vi "lorentzian from circle corners V5.vi"(7 "update z(inf)":enum16{"update z(inf)", "do not update z(inf)"}(ring)=enum."do not update z(inf)", 8 "omega map rameters in":T5={"frequency map method"=enum."less trivial", "2:window factor"=1, "left"=3.0, "right"=3.0, "omega"=3.0, "gamma"=3.0, "phi0"=3.0, "use points"=enum."decimated"}, 9 "circle corners in":T3={"z (-pi/2)"=-1.0311345636926572+0.5736824521422934i, "z(inf)"=-0.5200164984937075+1.0975277942502903i, "z (pi/2)"=-1.0311345636926572+0.5736824521422934i, "z center"=-0.5136528600391839+0.580046090596817i, "z(0)"=-0.5200164984937075+1.0975277942502903i, "radius"=-1.0311345636926572}, 10 "single fit parameters":T4={"number of 2D grid points"=200, "points after decimate"=93, "points before decimate"=4107, "decimation threshold"=1, "normalization factor"=0.005102552585135461, "complex region scale factor "=3.0, "normalized z"=array[4107 elements], "decimated z"=[0.4086999416726234+0.27653084474993667i, 0.4043675507393041+0.27187411611263035i, 0.3992152446406012+0.2866690148407477i, 0.38987681782092737+0.2796656705890701i, 0.3885478852115913+0.2853795752756981i, 0.37424677933088596+0.2916882969614883i, 0.36630586164105544+0.3013059695755191i, 0.3572225626966358+0.30157620929133466i, 0.3591607134412589+0.29870858500022546i, 0.34526037877213844+0.31577462619112134i, 0.3445358699361499+0.31396964671575356i, 0.34153004285372884+0.3154426636204338i, 0.335540381789013+0.3324302726540888i, 0.3288084132766795+0.33071696133989303i, 0.31551809708239975+0.34888246168069326i, 0.31398233630231437+0.34672841403398275i, 0.3124324305476661+0.34491167614050133i, 0.30168334846436345+0.36141080840589246i, 0.29960036161555575+0.3644765501140444i, 0.2787745634489416+0.3734961799530281i, 0.28247402044526565+0.37556030547495095i, 0.2654426354393931+0.38646722616569107i, 0.26085737469193576+0.39138156461276274i, 0.25158048144751116+0.4029098233705838i, 0.2437503606544421+0.40592983109982583i, 0.23659257658410568+0.4136463545042213i, 0.2208696574903446+0.4218755314447385i, 0.2037668036192148+0.4366037031685101i, 0.19187442018415896+0.438624011369513i, 0.17720511497204394+0.4432070269259341i, 0.1662607775835308+0.45453571196556497i, 0.1493802753732626+0.4639049582412799i, 0.1254511476775962+0.46748653333915113i, 0.1033303949534509+0.47813813399968913i, 0.0760179586599686+0.49136482745797033i, 0.03938352213850839+0.49341366586536217i, -0.008082261483109483+0.4963810216710412i, -0.060527992100659955+0.4985012896125286i, -0.13210308037505086+0.48328769389477994i, -0.2164964209072893+0.4579329803588853i, -0.31155150322000724+0.3898071876364797i, -0.41080908136967736+0.2764696089956603i, -0.47571311945822425+0.07542461980130123i, -0.43238189747242073-0.1750684238452788i, -0.2500583167802815-0.4029543655469544i, -0.003067977826097106-0.5014987103874714i, 0.19664864922046021-0.46877458226049556i, 0.3264592182464339-0.3841076764481272i, 0.39139158572573973-0.3045223037293669i, 0.4298267647472987-0.23258711184176573i, 0.4548604103609155-0.16798872385217029i, 0.46806747869399146-0.11764777517569555i, 0.47115569073873115-0.07926649929358924i, 0.46837628871708364-0.03694571328228424i, 0.47270651062714336-0.003809525374196055i, 0.47273283266207666+0.022081820056540025i, 0.4667717445305655+0.04127384443801294i, 0.46226887863084654+0.06320802982448562i, 0.4583729632879457+0.0875130923779392i, 0.4520889996996694+0.10406128252952807i, 0.45832267413717875+0.11311681771625329i, 0.4516869799167576+0.12298372020551539i, 0.4446055090004313+0.13178584688391243i, 0.44366854423885344+0.14231364306558697i, 0.4363006495505189+0.15757450828036026i, 0.42643994503455573+0.16593716221082852i, 0.42351872677287233+0.18339449448440692i, 0.41720623232577153+0.1988615890082908i, 0.41113704427571934+0.2125100714557952i, 0.40332364427545486+0.21990096302627865i, 0.4049190262834987+0.2293473262438519i, 0.39563214482126824+0.2405824404108469i, 0.38970786326899837+0.23506354711018443i, 0.3899681508881921+0.24823254471928627i, 0.3859413642570831+0.2582459848210299i, 0.3749803175874859+0.26059699274280157i, 0.3738379694867003+0.2718717578317005i, 0.35827051260491116+0.278162192718538i, 0.34435024044548757+0.2904452656920766i, 0.3297983655271314+0.29946214288730544i, 0.3299532953040057+0.30170168613834203i, 0.3258372999664237+0.31568274442045086i, 0.314591109715885+0.31037433654935476i, 0.31309403813828984+0.31627103049926253i, 0.29999544340655704+0.32049208568773396i, 0.29938213309261735+0.3149537822739577i, 0.28417087915090317+0.32544691504728024i, 0.29058669132467924+0.33251923664556715i, 0.2826528975116781+0.33032835058892424i, 0.2688413815997774+0.32858284064475973i, 0.2698123346444453+0.33078816617434537i, 0.25412663124852986+0.33157104396518056i, 0.2536781441982096+0.32875576565267184i], "decimated omega"=[2044.092, 2044.152, 2049.044, 2049.226, 2050.635, 2055.528, 2059.695, 2061.97, 2062.494, 2065.051, 2065.594, 2065.634, 2066.48, 2066.641, 2067.003, 2067.024, 2067.044, 2067.225, 2067.245, 2067.386, 2067.406, 2067.467, 2067.527, 2067.567, 2067.587, 2067.607, 2067.648, 2067.688, 2067.708, 2067.728, 2067.748, 2067.769, 2067.789, 2067.809, 2067.829, 2067.849, 2067.869, 2067.889, 2067.909, 2067.93, 2067.95, 2067.97, 2067.99, 2068.01, 2068.03, 2068.05, 2068.071, 2068.091, 2068.111, 2068.131, 2068.151, 2068.171, 2068.191, 2068.211, 2068.232, 2068.252, 2068.272, 2068.292, 2068.332, 2068.352, 2068.373, 2068.393, 2068.413, 2068.433, 2068.473, 2068.513, 2068.594, 2068.675, 2068.755, 2068.876, 2068.896, 2069.097, 2069.138, 2069.319, 2069.5, 2070.003, 2070.305, 2072.097, 2076.99, 2083.956, 2084.298, 2088.204, 2092.07, 2093.237, 2099.136, 2101.653, 2106.988, 2108.257, 2109.545, 2114.699, 2115.505, 2119.934, 2121.464], "omega in window"=array[4107 elements], "z in window"=array[4107 elements], "data center"=-0.0014901433980738042-0.0014987103874714112i, "inverse"=[], "linear "=[], "omega around"=[], "whatever plot"=[]}, 11 "cursor window":T1={"left"=2378.60310421286, "right "=2421.6740576496672, "center"=2421.6740576496672, "window"=2421.6740576496672, "cursors"=[], "relative"=0, "absolute"=0, "plot ref"=refnum, "Cursor List"=[], "fixed vertical offset"=2421.6740576496672, "vertical offset"=2421.6740576496672, "horizontal offset"=2421.6740576496672, "default window frac"=2421.6740576496672}) -> (0 "omega map rameters  out":T5={"frequency map method"=enum."less trivial", "2:window factor"=1, "left"=3.0, "right"=3.0, "omega"=3.0, "gamma"=3.0, "phi0"=3.0, "use points"=enum."decimated"}, 1 "circle corners out":T3={"z (-pi/2)"=-1.0311345636926572+0.5736824521422934i, "z(inf)"=-0.5200164984937075+1.0975277942502903i, "z (pi/2)"=-1.0311345636926572+0.5736824521422934i, "z center"=-0.5136528600391839+0.580046090596817i, "z(0)"=-0.5200164984937075+1.0975277942502903i, "radius"=-1.0311345636926572}, 3 "lorentzian out":T6={"Amplitude"=-1.0311345636926572, "omega(0)"=-1.0311345636926572, "Gamma"=-1.0311345636926572, "phi"=-1.0311345636926572, "Q"=-1.0311345636926572, "Norm  Ampl"=-1.0311345636926572, "z (inf)"=-1.0311345636926572+0.0i})   [LabVIEW 2010]
uses:
  <vilib>/Analysis/NI_AALPro.lvlib
  <vilib>/gmath/NI_Gmath.lvlib
  <vilib>/gmath/NumericalOptimization/Nonlinear Curve Fit LM.vi
  <vilib>/gmath/NumericalOptimization/LM model function reference.ctl
  <vilib>/Analysis/6fits.llb/Curve Fitting Criteria.ctl
  <vilib>/gmath/NumericalOptimization/Nonlinear Curve Fit LM formula string.vi
  circle corners.ctl
  lorentzian.ctl
  omega map parameters.ctl
  single fit parameters.ctl
  cursor winow.ctl
  <vilib>/Utility/miscctls.llb/LVCursorListTypeDef.ctl
panel:
  in  "lorentzian dummy 3":T6={"Amplitude"=-1.0311345636926572, "omega(0)"=-1.0311345636926572, "Gamma"=-1.0311345636926572, "phi"=-1.0311345636926572, "Q"=-1.0311345636926572, "Norm  Ampl"=-1.0311345636926572, "z (inf)"=-1.0311345636926572+0.0i}
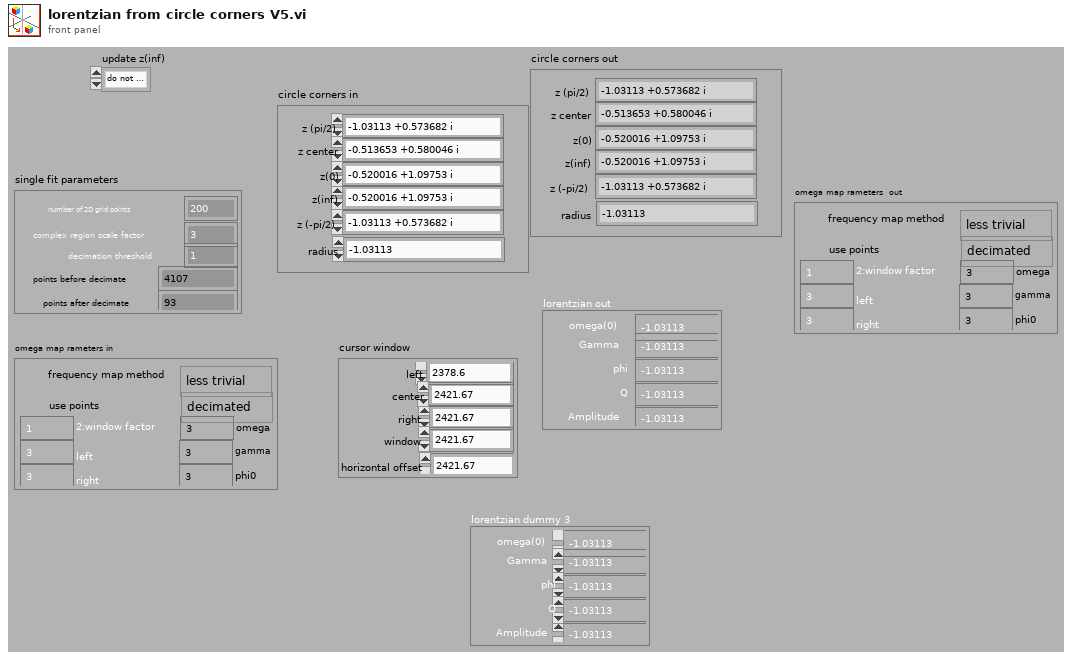
[diagram p1: front panel]
types:
  T1 = typedef "cursor winow.ctl" = cluster{"left":dbl, "right ":dbl, "center":dbl, "window":dbl, "cursors":i32[], "relative":i32, "absolute":i32, "plot ref":refnum<vi>, "Cursor List":T2, "fixed vertical offset":dbl, "vertical offset":dbl, "horizontal offset":dbl, "default window frac":dbl}
  T2 = typedef "LVCursorListTypeDef.ctl" = cluster{"Name":string, "Color":u32, "Style":u8, "Point Style":u8, "Name Visible":bool, "Allow Drag":bool, "Cursor Mode":u32, "Plot":i32, "Index":i32, "Position":cluster{"X":dbl, "Y":dbl}, "X Scale":u32, "Y Scale":u32, "Watch Plots":i32[], "Watch All Plots":bool, "Plot Area":i32, "Label Offset":cluster{"X":dbl, "Y":dbl}}[]
  T3 = typedef "circle corners.ctl" = cluster{"z (-pi/2)":cdb, "z(inf)":cdb, "z (pi/2)":cdb, "z center":cdb, "z(0)":cdb, "radius":dbl}
  T4 = typedef "single fit parameters.ctl" = cluster{"number of 2D grid points":i32, "points after decimate":i32, "points before decimate":i32, "decimation threshold":i32, "normalization factor":dbl, "complex region scale factor ":dbl, "normalized z":cdb[], "decimated z":cdb[], "decimated omega":dbl[], "omega in window":dbl[], "z in window":cdb[], "data center":cdb, "inverse":cdb[], "linear ":cdb[], "omega around":dbl[], "whatever plot":cluster{"omega":dbl[], dbl[]}[]}
  T5 = typedef "omega map parameters.ctl" = cluster{"frequency map method":enum16{"simple", "less trivial", "super fancy", "geometry"}, "2:window factor":i32, "left":dbl, "right":dbl, "omega":dbl, "gamma":dbl, "phi0":dbl, "use points":enum16{"all in window", "decimated"}}
  T6 = typedef "lorentzian.ctl" = cluster{"Amplitude":dbl, "omega(0)":dbl, "Gamma":dbl, "phi":dbl, "Q":dbl, "Norm  Ampl":dbl, "z (inf)":cdb}
  T7 = enum16{"simple method one", "not so simple method two", "super method three"}
  T8 = enum16{"simple", "less trivial", "super fancy", "geometry"}
  T9 = typedef "NI_Gmath.lvlib/LM model function reference.ctl" = refnum<vi>
  T10 = cluster{"model":string, "Parameters":string[], "x":string}
  T11 = cluster{"decimated omega":dbl[], "Unwrapped Phase":dbl[]}
  T12 = cluster{"decimated omega":dbl[], "best nonlinear fit":dbl[]}
  T13 = cluster{"decimated omega":dbl[], "best nonlinear fit":dbl[]}[]
  T14 = typedef "NI_AALPro.lvlib/Curve Fitting Criteria.ctl" = u16
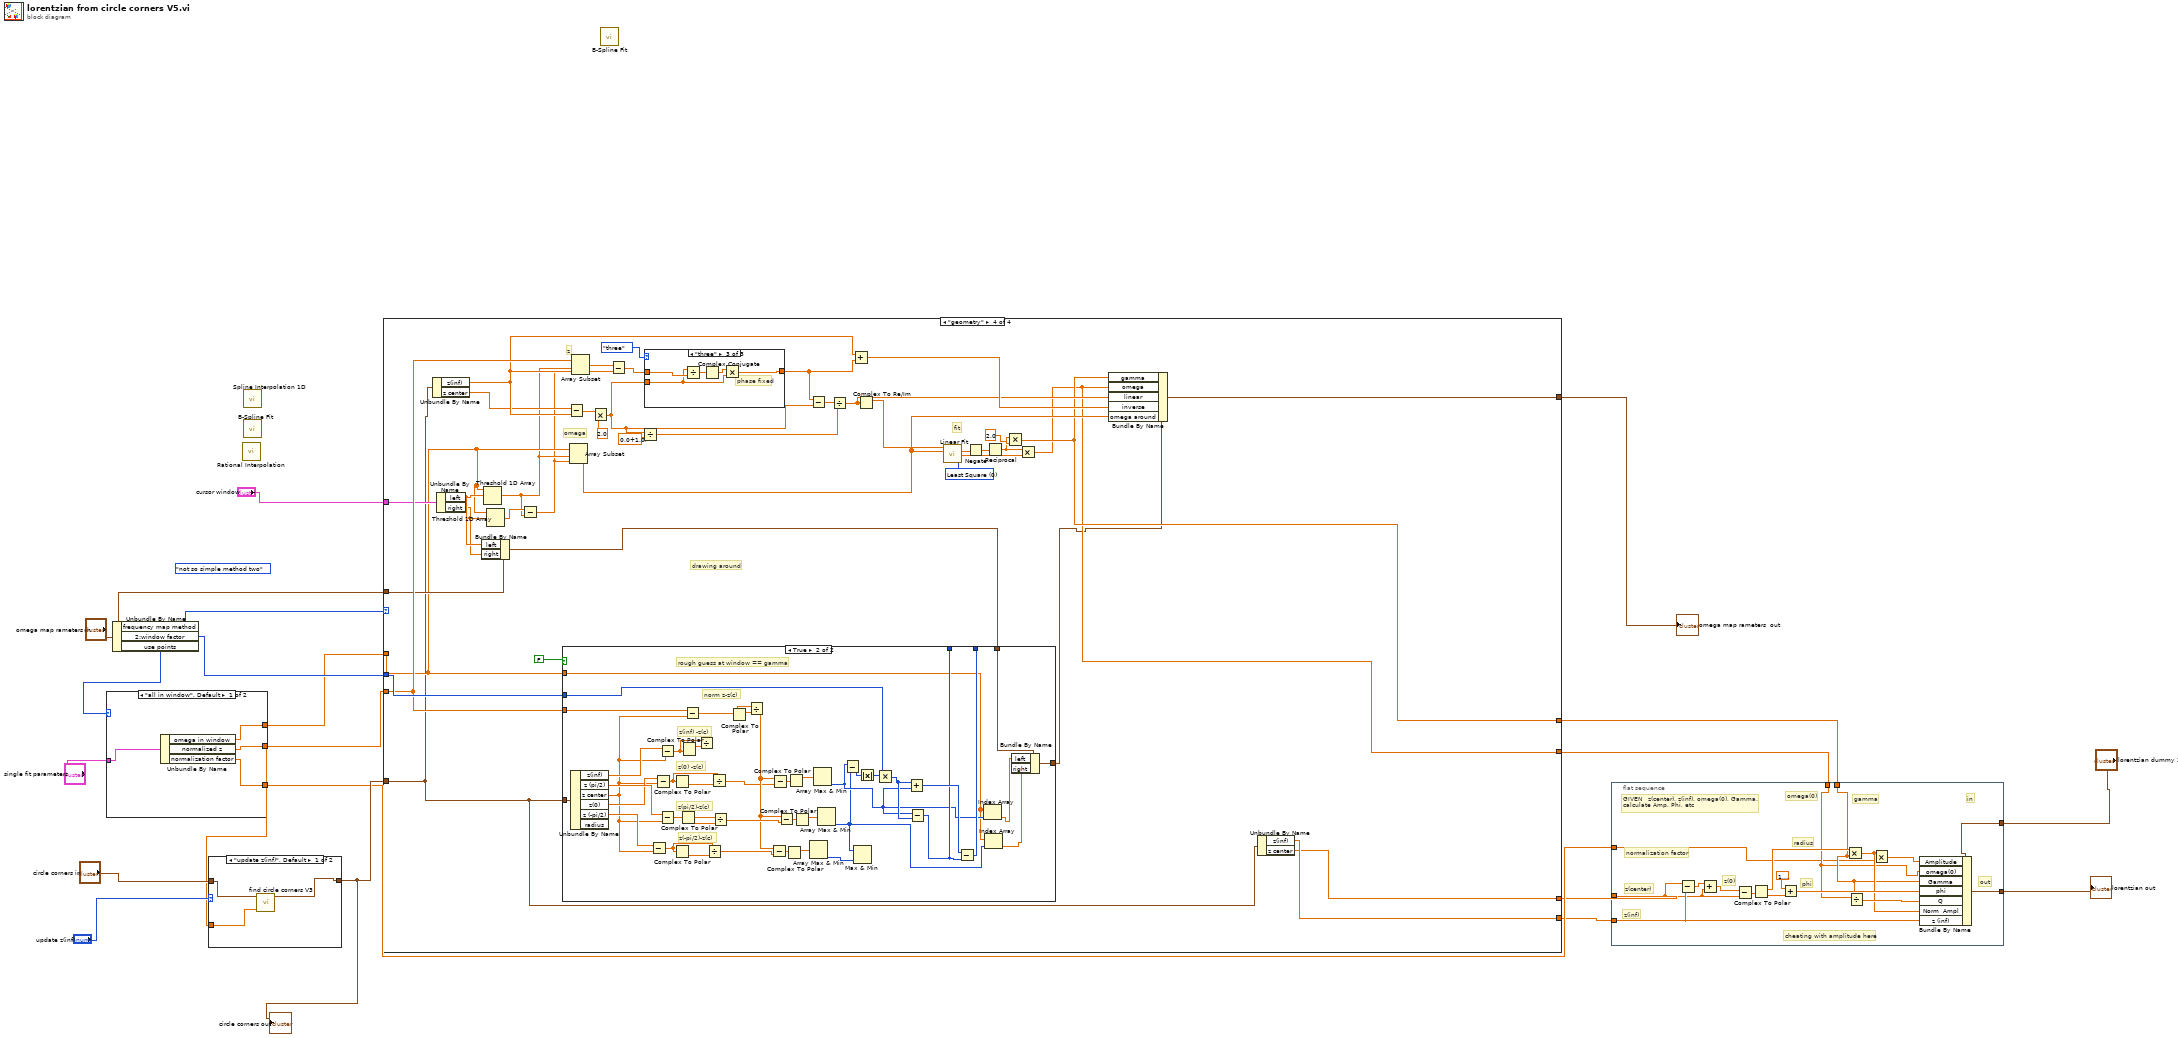
[diagram p0: block diagram]
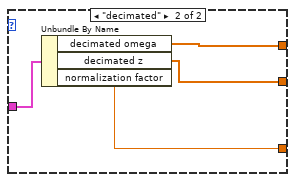
[diagram p3: hidden frame]
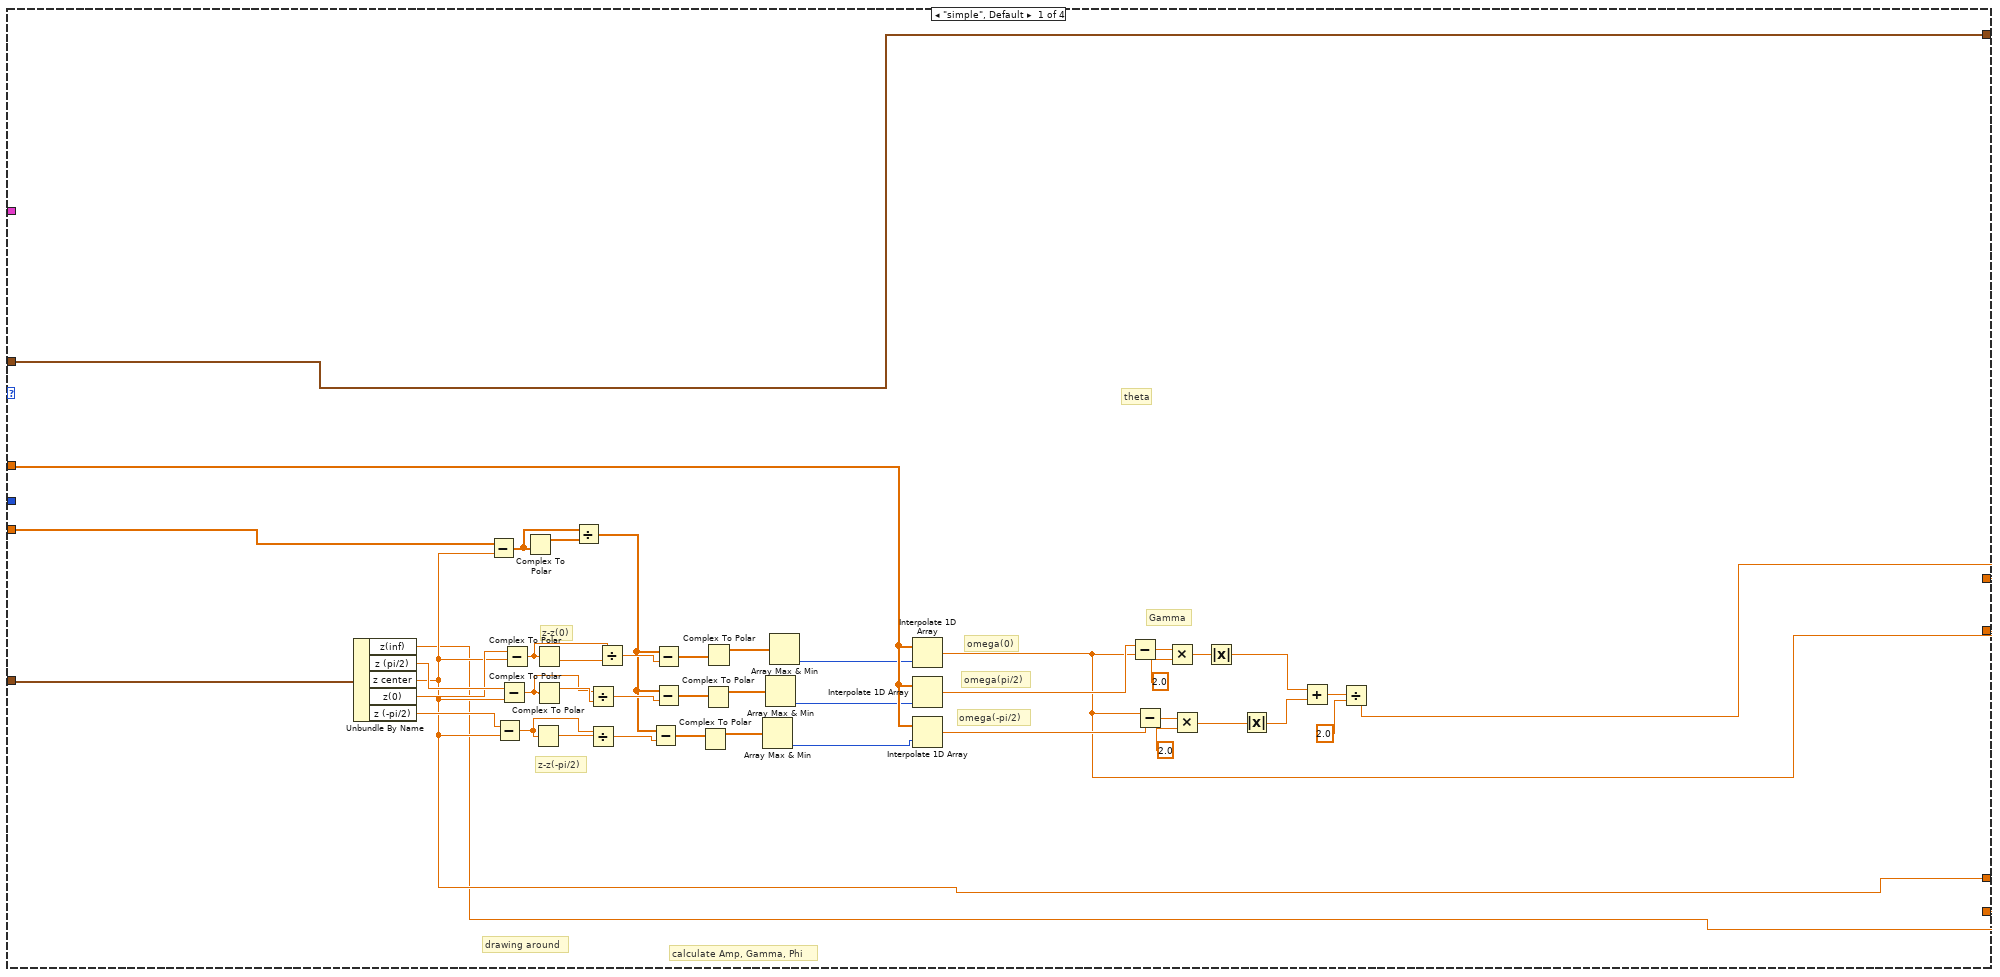
[diagram p4: hidden frame]
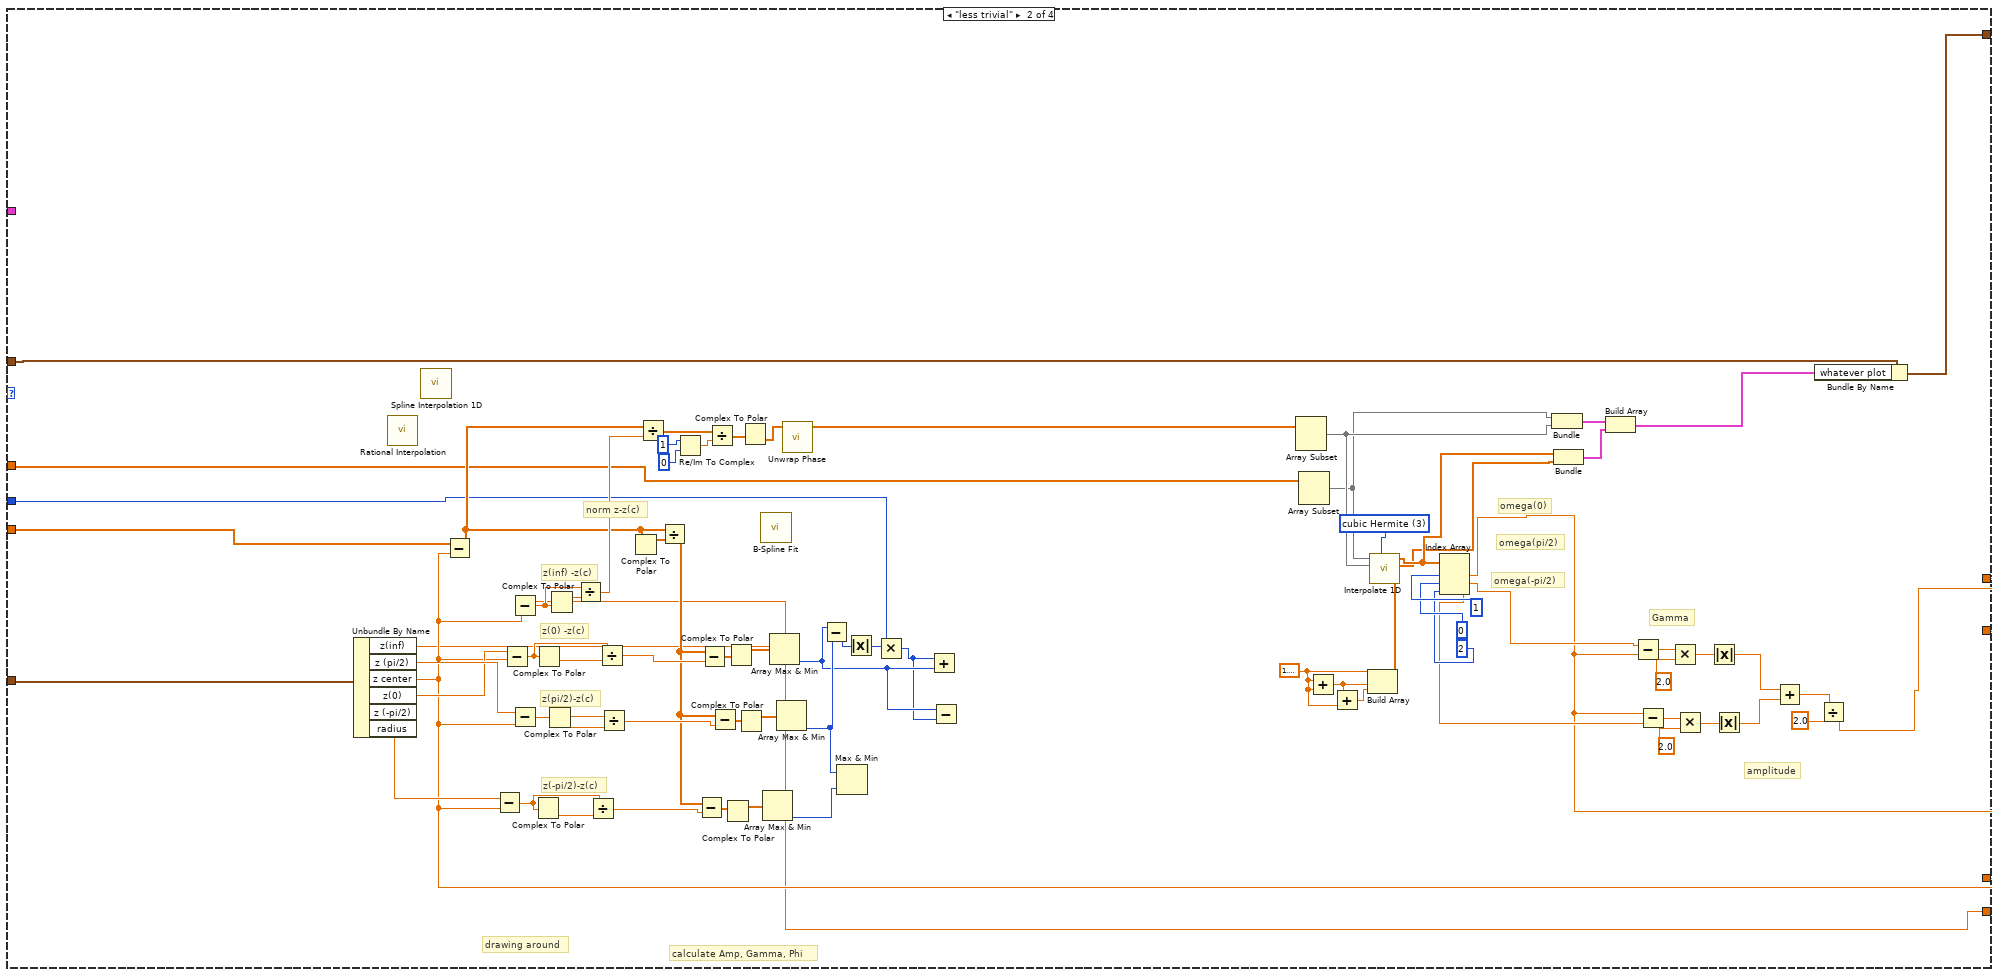
[diagram p5: hidden frame]
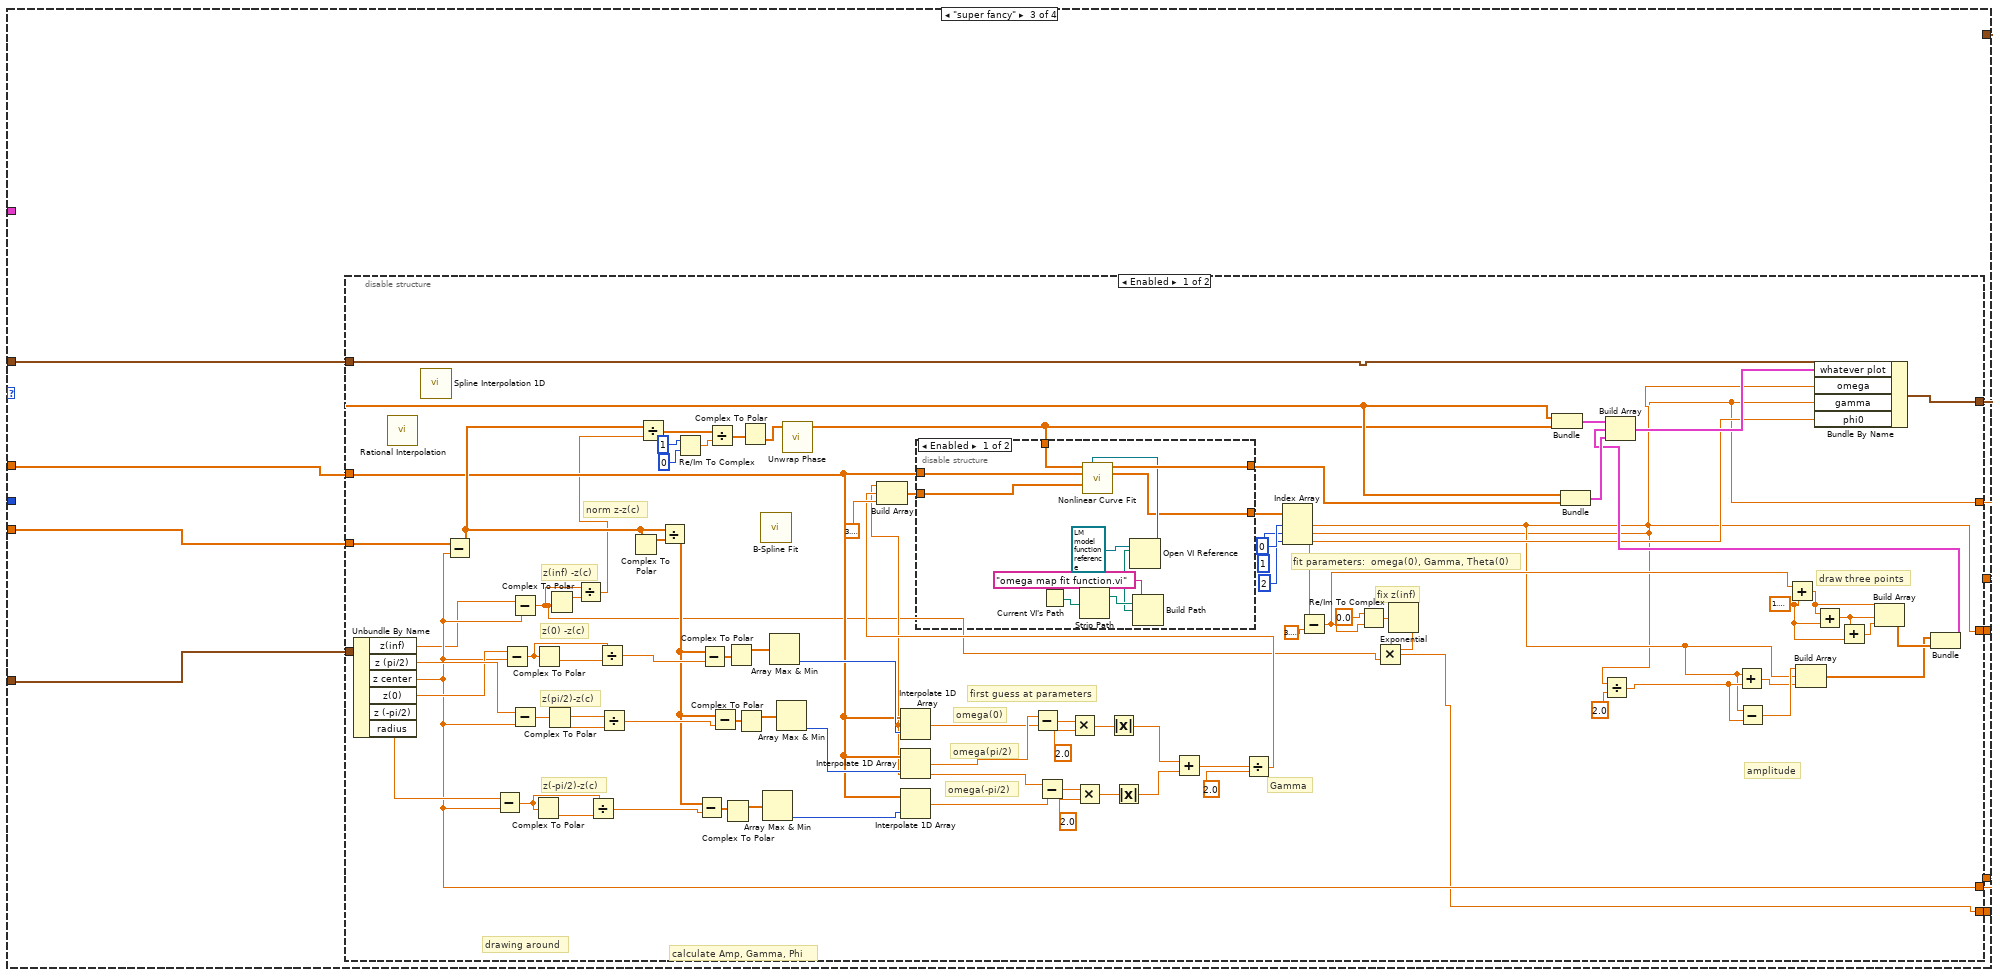
[diagram p6: hidden frame]
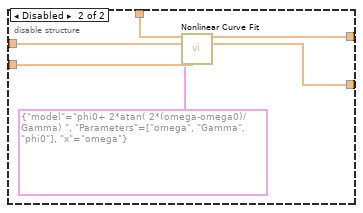
[diagram p7: hidden frame]
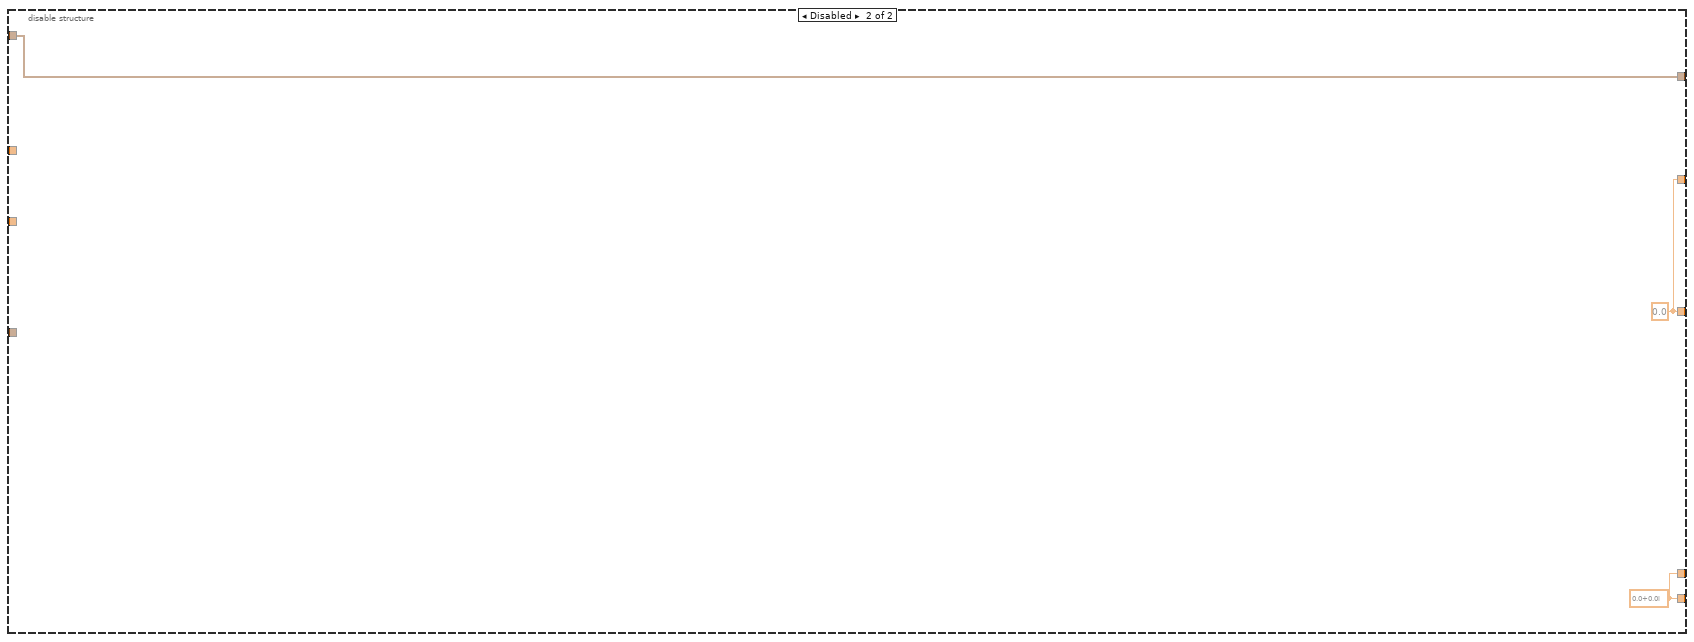
[diagram p8: hidden frame]
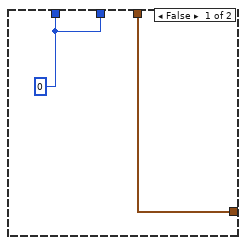
[diagram p9: hidden frame]
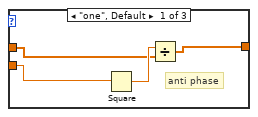
[diagram p10: hidden frame]
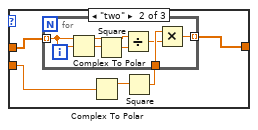
[diagram p11: hidden frame]
diagram:
  (unwired) T7."not so simple method two"
  n1 = Unbundle By Name("omega map rameters in") -> ("frequency map method"=w19:T8, "2:window factor"=w16:i32, "use points"=w13:enum16{"all in window", "decimated"})
  n2 = case shown="\"all in window\", Default" w13 {
    tunnel: "single fit parameters" -> [w23 w27]
    tunnel: [w22 w26] -> w14
    tunnel: [w21 w25] -> w10
    tunnel: [w20 w24] -> w4
    frame "all in window", Default {
      n3 = Unbundle By Name(w23) -> ("omega in window"=w22:dbl[], "normalized z"=w21:cdb[], "normalization factor"=w20:dbl)
    }
    frame "decimated" {
      n4 = Unbundle By Name(w27) -> ("decimated omega"=w26:dbl[], "decimated z"=w25:cdb[], "normalization factor"=w24:dbl)
    }
  }
  n5 = case shown="\"update z(inf)\", Default" "update z(inf)" {
    tunnel: [w29 w31] -> w9
    tunnel: "circle corners in" -> [w30 w31]
    tunnel: w10 -> [w28 _]
    frame "update z(inf)", Default {
      n6 = call "find circle corners V3.vi"("z"=w28, "circle corners in"=w30) -> ("circle corners out"=w29:T3)  [unwired: 9 in]
    }
    frame "do not update z(inf)" {
    }
  }
  "circle corners out" <- w9
  n7 = call <vilib>:"Rational Interpolation.vi"() -> ()  [unwired: 3 in, 3 out]
  n8 = call <vilib>:"Spline Interpolation 1D.vi"() -> ()  [unwired: 9 in, 3 out]
  n9 = call <vilib>:"B-Spline Fit.vi"() -> ()  [unwired: 12 in, 4 out]
  n10 = case shown="\"geometry\"" w19 {
    tunnel: w9 -> [w71 w146 w158 w264]
    tunnel: w10 -> [w70 w145 w157 w297]
    tunnel: w14 -> [w59 w105 w155 w270]
    tunnel: "omega map rameters in" -> [w36 w80 w154 w275]
    tunnel: [w36 w87 w156 w304] -> w17
    tunnel: w16 -> [_ w86 _ w303]
    tunnel: [w34 w78 w152 w281] -> w6
    tunnel: [w35 w79 w153 w280] -> w5
    tunnel: [w33 w77 w151 w265] -> w3
    tunnel: [w32 w76 w150 w266] -> w2
    tunnel: "cursor window" -> [_ _ _ w277]
    frame "simple", Default {
      # "z-z(-pi/2)"
      # "z-z(0)"
      # "omega(-pi/2)"
      # "omega(pi/2)"
      # "omega(0)"
      # "theta"
      # "Gamma"
      # "calculate Amp, Gamma, Phi"
      # "drawing around"
      n11 = Unbundle By Name(w71) -> ("z(inf)"=w32:cdb, "z (pi/2)"=w69:cdb, "z center"=w33:cdb, "z(0)"=w68:cdb, "z (-pi/2)"=w67:cdb)
      n12 = Subtract(x=w70, y=w33) -> (x-y=w51:cdb[])
      n13 = Subtract(x=w67, y=w33) -> (x-y=w54:cdb)
      n14 = Subtract(x=w69, y=w33) -> (x-y=w53:cdb)
      n15 = Subtract(x=w68, y=w33) -> (x-y=w58:cdb)
      n16 = Complex To Polar(r * e^(i*theta)=w51) -> (r=w52:dbl[])  [unwired: 1 out]
      n17 = Complex To Polar(r * e^(i*theta)=w54) -> (r=w56:dbl)  [unwired: 1 out]
      n18 = Complex To Polar(r * e^(i*theta)=w58) -> (r=w57:dbl)  [unwired: 1 out]
      n19 = Complex To Polar(r * e^(i*theta)=w53) -> (r=w55:dbl)  [unwired: 1 out]
      n20 = Divide(x=w51, y=w52) -> (x/y=w47:cdb[])
      n21 = Divide(x=w53, y=w55) -> (x/y=w49:cdb)
      n22 = Divide(x=w54, y=w56) -> (x/y=w48:cdb)
      n23 = Divide(x=w58, y=w57) -> (x/y=w50:cdb)
      n24 = Subtract(x=w47, y=w48) -> (x-y=w45:cdb[])
      n25 = Subtract(x=w47, y=w50) -> (x-y=w46:cdb[])
      n26 = Subtract(x=w47, y=w49) -> (x-y=w44:cdb[])
      n27 = Complex To Polar(r * e^(i*theta)=w45) -> (r=w41:dbl[])  [unwired: 1 out]
      n28 = Complex To Polar(r * e^(i*theta)=w44) -> (r=w42:dbl[])  [unwired: 1 out]
      n29 = Complex To Polar(r * e^(i*theta)=w46) -> (r=w43:dbl[])  [unwired: 1 out]
      n30 = Array Max & Min(array=w41) -> (min index (indices)=w40:i32)  [unwired: 3 out]
      n31 = Array Max & Min(array=w42) -> (min index (indices)=w39:i32)  [unwired: 3 out]
      n32 = Array Max & Min(array=w43) -> (min index (indices)=w38:i32)  [unwired: 3 out]
      n33 = Interpolate 1D Array(1:w38, 2:w59) -> (0:w35:dbl)
      n34 = Interpolate 1D Array(1:w39, 2:w59) -> (0:w72:dbl)
      n35 = Interpolate 1D Array(1:w40, 2:w59) -> (0:w60:dbl)
      n36 = Subtract(x=w72, y=w35) -> (x-y=w75:dbl)
      n37 = Subtract(x=w35, y=w60) -> (x-y=w66:dbl)
      n38 = Multiply(x=w75, y=2.0) -> (x*y=w73:dbl)
      n39 = Multiply(x=w66, y=2.0) -> (x*y=w64:dbl)
      n40 = Absolute Value(x=w73) -> (abs(x)=w63:dbl)
      n41 = Absolute Value(x=w64) -> (abs(x)=w37:dbl)
      n42 = Add(x=w63, y=w37) -> (x+y=w62:dbl)
      n43 = Divide(x=w62, y=2.0) -> (x/y=w34:dbl)
    }
    frame "less trivial" {
      w101 = 1.5707963267948966
      w103 = 3 items=["nearest", "linear", "spline", "cubic Hermite", "Lagrange"] ("method")
      # "z(pi/2)-z(c)"
      # "z(inf) -z(c)"
      # "norm z-z(c)"
      # "z(-pi/2)-z(c)"
      # "z(0) -z(c)"
      # "omega(-pi/2)"
      # "omega(pi/2)"
      # "omega(0)"
      # "amplitude"
      # "Gamma"
      # "calculate Amp, Gamma, Phi"
      # "drawing around"
      n44 = Unbundle By Name(w146) -> ("z(inf)"=w76:cdb, "z (pi/2)"=w144:cdb, "z center"=w77:cdb, "z(0)"=w143:cdb, "z (-pi/2)"=w142:cdb)  [unwired: 1 out]
      n45 = call <vilib>:"Rational Interpolation.vi"() -> ()  [unwired: 3 in, 3 out]
      n46 = call <vilib>:"Spline Interpolation 1D.vi"() -> ()  [unwired: 9 in, 3 out]
      n47 = Subtract(x=w145, y=w77) -> (x-y=w114:cdb[])
      n48 = Subtract(x=w142, y=w77) -> (x-y=w132:cdb)
      n49 = Subtract(x=w143, y=w77) -> (x-y=w135:cdb)
      n50 = Subtract(x=w76, y=w77) -> (x-y=w118:cdb)
      n51 = Subtract(x=w144, y=w77) -> (x-y=w131:cdb)
      n52 = Complex To Polar(r * e^(i*theta)=w132) -> (r=w133:dbl)  [unwired: 1 out]
      n53 = Complex To Polar(r * e^(i*theta)=w135) -> (r=w134:dbl)  [unwired: 1 out]
      n54 = Complex To Polar(r * e^(i*theta)=w131) -> (r=w107:dbl)  [unwired: 1 out]
      n55 = Complex To Polar(r * e^(i*theta)=w118) -> (r=w119:dbl)  [unwired: 1 out]
      n56 = Divide(x=w118, y=w119) -> (x/y=w117:cdb)
      n57 = Divide(x=w132, y=w133) -> (x/y=w127:cdb)
      n58 = Divide(x=w135, y=w134) -> (x/y=w129:cdb)
      n59 = Divide(x=w131, y=w107) -> (x/y=w128:cdb)
      n60 = Complex To Polar(r * e^(i*theta)=w114) -> (r=w130:dbl[])  [unwired: 1 out]
      n61 = Divide(x=w114, y=w117) -> (x/y=w110:cdb[])
      n62 = Divide(x=w114, y=w130) -> (x/y=w116:cdb[])
      n63 = Re/Im To Complex(1:0, 2:1) -> (0:w112:cdb)
      n64 = Subtract(x=w116, y=w127) -> (x-y=w125:cdb[])
      n65 = Subtract(x=w116, y=w129) -> (x-y=w126:cdb[])
      n66 = Divide(x=w110, y=w112) -> (x/y=w113:cdb[])
      n67 = Subtract(x=w116, y=w128) -> (x-y=w124:cdb[])
      n68 = Complex To Polar(r * e^(i*theta)=w125) -> (r=w121:dbl[])  [unwired: 1 out]
      n69 = Complex To Polar(r * e^(i*theta)=w126) -> (r=w123:dbl[])  [unwired: 1 out]
      n70 = Complex To Polar(r * e^(i*theta)=w124) -> (r=w122:dbl[])  [unwired: 1 out]
      n71 = Complex To Polar(r * e^(i*theta)=w113) -> (theta=w108:dbl[])  [unwired: 1 out]
      n72 = call <vilib>:"B-Spline Fit.vi"() -> ()  [unwired: 12 in, 4 out]
      n73 = Array Max & Min(array=w121) -> (min index (indices)=w106:i32)  [unwired: 3 out]
      n74 = Array Max & Min(array=w123) -> (min index (indices)=w90:i32)  [unwired: 3 out]
      n75 = Array Max & Min(array=w122) -> (min index (indices)=w93:i32)  [unwired: 3 out]
      n76 = call <vilib>:"Unwrap Phase.vi"("Phase"=w108) -> ("Unwrapped Phase"=w104:dbl[])  [unwired: 9 in, 1 out]
      n77 = Subtract(x=w90, y=w93) -> (x-y=w92:i32)
      n78 = Max & Min(x=w93, y=w106) -> ()  [unwired: 2 out]
      n79 = Absolute Value(x=w92) -> (abs(x)=w91:i32)
      n80 = Multiply(x=w91, y=w86) -> (x*y=w89:i32)
      n81 = Add(x=w89, y=w90) -> ()  [unwired: 1 out]
      n82 = Subtract(x=w90, y=w89) -> ()  [unwired: 1 out]
      n83 = Array Subset(array=w104) -> (w95:dbl[])  [unwired: 2 in]
      n84 = Array Subset(array=w105) -> (w94:dbl[])  [unwired: 2 in]
      n85 = Add(x=w101, y=w101) -> (x+y=w102:dbl)
      n86 = Add(x=w102, y=w101) -> (x+y=w100:dbl)
      n87 = Build Array(w101, w102, w100) -> (w99:dbl[])
      n88 = call <vilib>:"Interpolate 1D.vi"("method"=w103, "xi"=w99, "X"=w95, "Y"=w94) -> ("xi used"=w84:dbl[], "yi"=w85:dbl[])  [unwired: 5 in, 1 out]
      n89 = Index Array(array=w85, index #1=1, index #2=0, index #3=2) -> (element #1=w79:dbl, element #2=w82:dbl, element #3=w81:dbl)
      n90 = Bundle(w94, w95) -> (w115:cluster{dbl[], dbl[]})  [unwired: 1 in]
      n91 = Bundle("yi"=w85, "xi used"=w84) -> (w83:cluster{"yi":dbl[], "xi used":dbl[]})  [unwired: 1 in]
      n92 = Build Array(w115, w83) -> (w88:cluster{"yi":dbl[], "xi used":dbl[]}[])
      n93 = Subtract(x=w82, y=w79) -> (x-y=w149:dbl)
      n94 = Subtract(x=w79, y=w81) -> (x-y=w141:dbl)
      n95 = Multiply(x=w149, y=2.0) -> (x*y=w147:dbl)
      n96 = Multiply(x=w141, y=2.0) -> (x*y=w139:dbl)
      n97 = Absolute Value(x=w147) -> (abs(x)=w138:dbl)
      n98 = Absolute Value(x=w139) -> (abs(x)=w120:dbl)
      n99 = Add(x=w138, y=w120) -> (x+y=w137:dbl)
      n100 = Bundle By Name(cluster=w80, "whatever plot"=w88) -> (w87:T5)
      n101 = Divide(x=w137, y=2.0) -> (x/y=w78:dbl)
    }
    frame "super fancy" {
      n102 = disable-structure shown="Enabled" {
        disable-tunnel: w158 -> [w243 _]
        disable-tunnel: w157 -> [w242 _]
        disable-tunnel: [w211 w263] -> w156
        disable-tunnel: w155 -> [w193 _]
        disable-tunnel: w154 -> [w191 w263]
        disable-tunnel: [w163 w261] -> w153
        disable-tunnel: [w162 w261] -> w152
        disable-tunnel: [w161 w262] -> w151
        disable-tunnel: [w159 w262] -> w150
        frame Enabled {
          w167 = 1.5707963267948966
          # "fix z(inf)"
          # "fit parameters:  omega(0), Gamma, Theta(0)"
          # "draw three points"
          # "first guess at parameters"
          # "omega(-pi/2)"
          # "omega(pi/2)"
          # "omega(0)"
          # "Gamma"
          # "z(pi/2)-z(c)"
          # "z(inf) -z(c)"
          # "norm z-z(c)"
          # "z(-pi/2)-z(c)"
          # "z(0) -z(c)"
          # "amplitude"
          # "calculate Amp, Gamma, Phi"
          # "drawing around"
          n103 = Unbundle By Name(w243) -> ("z(inf)"=w160:cdb, "z (pi/2)"=w241:cdb, "z center"=w161:cdb, "z(0)"=w240:cdb, "z (-pi/2)"=w239:cdb)  [unwired: 1 out]
          n104 = call <vilib>:"Rational Interpolation.vi"() -> ()  [unwired: 3 in, 3 out]
          n105 = call <vilib>:"Spline Interpolation 1D.vi"() -> ()  [unwired: 9 in, 3 out]
          n106 = Subtract(x=w242, y=w161) -> (x-y=w220:cdb[])
          n107 = Subtract(x=w239, y=w161) -> (x-y=w235:cdb)
          n108 = Subtract(x=w240, y=w161) -> (x-y=w238:cdb)
          n109 = Subtract(x=w160, y=w161) -> (x-y=w166:cdb)
          n110 = Subtract(x=w241, y=w161) -> (x-y=w234:cdb)
          n111 = Complex To Polar(r * e^(i*theta)=w235) -> (r=w236:dbl)  [unwired: 1 out]
          n112 = Complex To Polar(r * e^(i*theta)=w238) -> (r=w237:dbl)  [unwired: 1 out]
          n113 = Complex To Polar(r * e^(i*theta)=w234) -> (r=w213:dbl)  [unwired: 1 out]
          n114 = Complex To Polar(r * e^(i*theta)=w166) -> (r=w223:dbl)  [unwired: 1 out]
          n115 = Divide(x=w166, y=w223) -> (x/y=w173:cdb)
          n116 = Divide(x=w235, y=w236) -> (x/y=w230:cdb)
          n117 = Divide(x=w238, y=w237) -> (x/y=w232:cdb)
          n118 = Divide(x=w234, y=w213) -> (x/y=w231:cdb)
          n119 = Complex To Polar(r * e^(i*theta)=w220) -> (r=w233:dbl[])  [unwired: 1 out]
          n120 = Divide(x=w220, y=w173) -> (x/y=w216:cdb[])
          n121 = Divide(x=w220, y=w233) -> (x/y=w222:cdb[])
          n122 = Re/Im To Complex(1:0, 2:1) -> (0:w218:cdb)
          n123 = Subtract(x=w222, y=w230) -> (x-y=w228:cdb[])
          n124 = Subtract(x=w222, y=w232) -> (x-y=w229:cdb[])
          n125 = Divide(x=w216, y=w218) -> (x/y=w219:cdb[])
          n126 = Subtract(x=w222, y=w231) -> (x-y=w227:cdb[])
          n127 = Complex To Polar(r * e^(i*theta)=w228) -> (r=w224:dbl[])  [unwired: 1 out]
          n128 = Complex To Polar(r * e^(i*theta)=w229) -> (r=w226:dbl[])  [unwired: 1 out]
          n129 = Complex To Polar(r * e^(i*theta)=w227) -> (r=w225:dbl[])  [unwired: 1 out]
          n130 = Complex To Polar(r * e^(i*theta)=w219) -> (theta=w214:dbl[])  [unwired: 1 out]
          n131 = call <vilib>:"B-Spline Fit.vi"() -> ()  [unwired: 12 in, 4 out]
          n132 = Array Max & Min(array=w224) -> (min index (indices)=w194:i32)  [unwired: 3 out]
          n133 = Array Max & Min(array=w226) -> (min index (indices)=w196:i32)  [unwired: 3 out]
          n134 = Array Max & Min(array=w225) -> (min index (indices)=w195:i32)  [unwired: 3 out]
          n135 = call <vilib>:"Unwrap Phase.vi"("Phase"=w214) -> ("Unwrapped Phase"=w192:dbl[])  [unwired: 9 in, 1 out]
          n136 = Interpolate 1D Array(1:w196, 2:w193) -> (0:w187:dbl)
          n137 = Interpolate 1D Array(1:w195, 2:w193) -> (0:w189:dbl)
          n138 = Interpolate 1D Array(1:w194, 2:w193) -> (0:w188:dbl)
          n139 = Subtract(x=w189, y=w187) -> (x-y=w206:dbl)
          n140 = Subtract(x=w187, y=w188) -> (x-y=w203:dbl)
          n141 = Multiply(x=w206, y=2.0) -> (x*y=w204:dbl)
          n142 = Multiply(x=w203, y=2.0) -> (x*y=w201:dbl)
          n143 = Absolute Value(x=w204) -> (abs(x)=w200:dbl)
          n144 = Absolute Value(x=w201) -> (abs(x)=w197:dbl)
          n145 = Add(x=w200, y=w197) -> (x+y=w199:dbl)
          n146 = Divide(x=w199, y=2.0) -> (x/y=w190:dbl)
          n147 = Build Array(w187, w190, 3.141592653589793) -> (w209:dbl[])
          n148 = disable-structure shown="Enabled" {
            disable-tunnel: w209 -> [w254 w260]
            disable-tunnel: [w253 w256] -> w208
            disable-tunnel: w193 -> [w246 w258]
            disable-tunnel: w192 -> [w245 w259]
            disable-tunnel: [w244 w255] -> w186
            frame Enabled {
              n149 = Current VI's Path() -> (path=w251:path)
              n150 = Strip Path(path=w251) -> (stripped path=w250:path)  [unwired: 1 out]
              n151 = Build Path(base path=w250, name or relative path="omega map fit function.vi" ("f(x,a) VI name Complex")) -> (appended path=w248:path)
              n152 = Open VI Reference(type specifier VI Refnum (for type only)=T9 refnum ("f(x,a)"), vi path=w248) -> (vi reference=w247:T9)  [unwired: 1 in, 4 out]
              n153 = call-poly <vilib>:"Nonlinear Curve Fit.vi"("Y"=w245, "f(x,a)"=w247, "X"=w246, "initial parameters"=w254) -> ("best nonlinear fit"=w253:dbl[], "best fit parameters"=w244:dbl[])  [unwired: 6 in, 4 out]
            }
            frame Disabled {
              n154 = call-poly <vilib>:"Nonlinear Curve Fit.vi"("Y"=w259, "initial parameters"=w260, "X"=w258, "model description"=T10 {"model"="phi0+ 2*atan( 2*(omega-omega0)/Gamma) ", "Parameters"=["omega", "Gamma", "phi0"], "x"="omega"}) -> ("best nonlinear fit"=w256:dbl[], "best fit parameters"=w255:dbl[])  [unwired: 7 in, 3 out]
            }
          }
          n155 = Index Array(array=w186, index #1=0, index #2=1, index #3=2) -> (element #1=w163:dbl, element #2=w162:dbl, element #3=w171:dbl)
          n156 = Subtract(x=w171, y=3.141592653589793) -> (x-y=w168:dbl)
          n157 = Re/Im To Complex(1:w168, 2:0.0) -> (0:w174:cdb)
          n158 = Exponential(1:w174) -> (0:w172:cdb)
          n159 = Multiply(x=w172, y=w166) -> (x*y=w159:cdb)
          n160 = Bundle("decimated omega"=w193, "Unwrapped Phase"=w192) -> (w221:T11)  [unwired: 1 in]
          n161 = Bundle("decimated omega"=w193, "best nonlinear fit"=w208) -> (w207:T12)  [unwired: 1 in]
          n162 = Divide(x=w162, y=2.0) -> (x/y=w164:dbl)
          n163 = Add(x=w163, y=w164) -> (x+y=w176:dbl)
          n164 = Subtract(x=w163, y=w164) -> (x-y=w177:dbl)
          n165 = Add(x=w168, y=w167) -> (x+y=w169:dbl)
          n166 = Build Array(w177, w163, w176) -> (w178:dbl[])
          n167 = Add(x=w169, y=w167) -> (x+y=w182:dbl)
          n168 = Add(x=w182, y=w167) -> (x+y=w181:dbl)
          n169 = Build Array(w169, w182, w181) -> (w179:dbl[])
          n170 = Bundle(w178, w179) -> (w180:cluster{dbl[], dbl[]})  [unwired: 1 in]
          n171 = Build Array(w221, w180, w207) -> (w212:T13)
          n172 = Bundle By Name(cluster=w191, "whatever plot"=w212, "omega"=w163, "gamma"=w162, "phi0"=w171) -> (w211:T5)
        }
        frame Disabled {
          w261 = 0.0 ("Numeric")
          w262 = cdb 0.0+0.0i
        }
      }
    }
    frame "geometry" {
      w291 = T14 0 items=["Least Square", "Least Absolute Residual", "Bisquare"] ("method")
      # "fit"
      # "z"
      # "omega"
      # "drawing around"
      n173 = Unbundle By Name(w264) -> ("z(inf)"=w279:cdb, "z center"=w278:cdb)
      n174 = Unbundle By Name(w277) -> ("left"=w274:dbl, "right"=w271:dbl)
      n175 = Bundle By Name(cluster=w275, "left"=w274, "right"=w271) -> (w273:T5)
      n176 = Threshold 1D Array(2:w274, 3:w270) -> (0:w268:dbl)  [unwired: 1 in]
      n177 = Threshold 1D Array(2:w271, 3:w270) -> (0:w269:dbl)  [unwired: 1 in]
      n178 = Subtract(x=w269, y=w268) -> (x-y=w267:dbl)
      n179 = case shown="True" FALSE {
        tunnel: w303 -> [_ w322]
        tunnel: w297 -> [_ w321]
        tunnel: [w305 w320] -> _
        tunnel: [w305 w319] -> _
        tunnel: w270 -> [_ w316]
        tunnel: w264 -> [_ w314]
        tunnel: [w306 w309] -> w272
        tunnel: w273 -> [w306 w308]
        frame False {
          w305 = 0
        }
        frame True {
          # "rough guess at window == gamma"
          # "z(pi/2)-z(c)"
          # "z(inf) -z(c)"
          # "norm z-z(c)"
          # "z(-pi/2)-z(c)"
          # "z(0) -z(c)"
          n180 = Unbundle By Name(w314) -> ("z(inf)"=w313:cdb, "z (pi/2)"=w348:cdb, "z center"=w312:cdb, "z(0)"=w347:cdb, "z (-pi/2)"=w315:cdb)  [unwired: 1 out]
          n181 = Subtract(x=w315, y=w312) -> (x-y=w343:cdb)
          n182 = Subtract(x=w347, y=w312) -> (x-y=w346:cdb)
          n183 = Subtract(x=w313, y=w312) -> (x-y=w331:cdb)
          n184 = Subtract(x=w348, y=w312) -> (x-y=w342:cdb)
          n185 = Complex To Polar(r * e^(i*theta)=w346) -> (r=w345:dbl)  [unwired: 1 out]
          n186 = Complex To Polar(r * e^(i*theta)=w343) -> (r=w344:dbl)  [unwired: 1 out]
          n187 = Complex To Polar(r * e^(i*theta)=w342) -> (r=w328:dbl)  [unwired: 1 out]
          n188 = Complex To Polar(r * e^(i*theta)=w331) -> (r=w332:dbl)  [unwired: 1 out]
          n189 = Subtract(x=w321, y=w312) -> (x-y=w329:cdb[])
          n190 = Divide(x=w331, y=w332) -> ()  [unwired: 1 out]
          n191 = Divide(x=w343, y=w344) -> (x/y=w339:cdb)
          n192 = Divide(x=w346, y=w345) -> (x/y=w307:cdb)
          n193 = Divide(x=w342, y=w328) -> (x/y=w340:cdb)
          n194 = Complex To Polar(r * e^(i*theta)=w329) -> (r=w341:dbl[])  [unwired: 1 out]
          n195 = Divide(x=w329, y=w341) -> (x/y=w330:cdb[])
          n196 = Subtract(x=w330, y=w339) -> (x-y=w337:cdb[])
          n197 = Subtract(x=w330, y=w307) -> (x-y=w338:cdb[])
          n198 = Subtract(x=w330, y=w340) -> (x-y=w336:cdb[])
          n199 = Complex To Polar(r * e^(i*theta)=w337) -> (r=w333:dbl[])  [unwired: 1 out]
          n200 = Complex To Polar(r * e^(i*theta)=w338) -> (r=w335:dbl[])  [unwired: 1 out]
          n201 = Complex To Polar(r * e^(i*theta)=w336) -> (r=w334:dbl[])  [unwired: 1 out]
          n202 = Array Max & Min(array=w333) -> (min index (indices)=w327:i32)  [unwired: 3 out]
          n203 = Array Max & Min(array=w335) -> (min index (indices)=w318:i32)  [unwired: 3 out]
          n204 = Array Max & Min(array=w334) -> (min index (indices)=w317:i32)  [unwired: 3 out]
          n205 = Subtract(x=w318, y=w317) -> (x-y=w326:i32)
          n206 = Max & Min(x=w317, y=w327) -> ()  [unwired: 2 out]
          n207 = Absolute Value(x=w326) -> (abs(x)=w325:i32)
          n208 = Multiply(x=w325, y=w322) -> (x*y=w324:i32)
          n209 = Add(x=w324, y=w318) -> (x+y=w323:i32)
          n210 = Subtract(x=w318, y=w324) -> (x-y=w319:i32)
          n211 = Subtract(x=w323, y=w319) -> (x-y=w320:i32)
          n212 = Index Array(array=w316, index=w318) -> (element=w311:dbl)
          n213 = Index Array(array=w316, index=w317) -> (element=w310:dbl)
          n214 = Bundle By Name(cluster=w308, "left"=w311, "right"=w310) -> (w309:T5)
        }
      }
      n215 = Subtract(x=w278, y=w279) -> (x-y=w301:cdb)
      n216 = Array Subset(array=w270, index=w268, length=w267) -> (w283:dbl[])
      n217 = Array Subset(array=w297, index=w268, length=w267) -> (w296:cdb[])
      n218 = Multiply(x=w301, y=2.0) -> (x*y=w295:cdb)
      n219 = Subtract(x=w296, y=w279) -> (x-y=w300:cdb[])
      n220 = Divide(x=w295, y=cdb 0.0+1.0i) -> (x/y=w293:cdb)
      n221 = case shown="\"three\"" enum16{"one", "three", "two"}."three" {
        tunnel: w300 -> [w350 w357 w368]
        tunnel: [w349 w354 w364] -> w299
        tunnel: w295 -> [w352 w353 w365]
        frame "one", Default {
          # "anti phase"
          n222 = Square(x=w352) -> (x^2=w351:cdb)
          n223 = Divide(x=w351, y=w350) -> (x/y=w349:cdb[])
        }
        frame "two" {
          n224 = Complex To Polar(r * e^(i*theta)=w353) -> (r=w356:dbl)  [unwired: 1 out]
          n225 = Square(x=w356) -> (x^2=w355:dbl)
          n226 = for {
            tunnel: w357 -> [w363] mode=indexing
            tunnel: w355 -> [w360]
            tunnel: [w358] -> w354 mode=indexing
            n227 = Complex To Polar(r * e^(i*theta)=w363) -> (r=w361:dbl)  [unwired: 1 out]
            n228 = Square(x=w361) -> (x^2=w362:dbl)
            n229 = Divide(x=w363, y=w362) -> (x/y=w359:cdb)
            n230 = Multiply(x=w360, y=w359) -> (x*y=w358:cdb)
          }
        }
        frame "three" {
          # "phase fixed"
          n231 = Divide(x=w365, y=w368) -> (x/y=w367:cdb[])
          n232 = Complex Conjugate(1:w367) -> (0:w366:cdb[])
          n233 = Multiply(x=w366, y=w365) -> (x*y=w364:cdb[])
        }
      }
      n234 = Subtract(x=w299, y=w295) -> (x-y=w298:cdb[])
      n235 = Divide(x=w298, y=w293) -> (x/y=w284:cdb[])
      n236 = Add(x=w279, y=w299) -> (x+y=w285:cdb[])
      n237 = Complex To Re/Im(x + iy=w284) -> (x=w292:dbl[])  [unwired: 1 out]
      n238 = call <vilib>:"Linear Fit.vi"("Y"=w292, "X"=w283, "method"=w291) -> ("slope"=w289:dbl, "intercept"=w287:dbl)  [unwired: 8 in, 3 out]
      n239 = Negate(x=w289) -> (-x=w288:dbl)
      n240 = Reciprocal(x=w288) -> (1/x=w286:dbl)
      n241 = Multiply(x=w286, y=2.0) -> (x*y=w281:dbl)
      n242 = Multiply(x=w286, y=w287) -> (x*y=w280:dbl)
      n243 = Bundle By Name(cluster=w272, "gamma"=w281, "omega"=w280, "linear"=w284, "inverse"=w285, "omega around"=w283) -> (w304:T5)
      n244 = Unbundle By Name(w264) -> ("z(inf)"=w266:cdb, "z center"=w265:cdb)
    }
  }
  "omega map rameters  out" <- w17
  n245 = call <vilib>:"B-Spline Fit.vi"() -> ()  [unwired: 12 in, 4 out]
  n246 = flat-sequence {
    tunnel: w2 -> [w377]
    tunnel: w3 -> [w375]
    tunnel: "lorentzian dummy 3" -> [w373]
    tunnel: [w372] -> w7
    tunnel: w6 -> [w371]
    tunnel: w5 -> [w370]
    tunnel: w4 -> [w369]
    frame #0 {
      # "out"
      # "in"
      # "GIVEN   z(center), z(inf), omega(0), Gamma, \ncalculate Amp, Phi, etc"
      # "z(center)"
      # "z(0)"
      # "z(inf)"
      # "normalization factor"
      # "radius"
      # "omega(0)"
      # "gamma"
      # "phi"
      # "cheating with amplitude here"
      n247 = Subtract(x=w375, y=w377) -> (x-y=w376:cdb)
      n248 = Add(x=w376, y=w375) -> (x+y=w374:cdb)
      n249 = Subtract(x=w374, y=w375) -> (x-y=w385:cdb)
      n250 = Complex To Polar(r * e^(i*theta)=w385) -> (r=w378:dbl, theta=w383:dbl)
      n251 = Add(x=1.5707963267948966, y=w383) -> (x+y=w382:dbl)
      n252 = Multiply(x=w378, y=w371) -> (x*y=w380:dbl)
      n253 = Divide(x=w370, y=w371) -> (x/y=w381:dbl)
      n254 = Multiply(x=w380, y=w369) -> (x*y=w379:dbl)
      n255 = Bundle By Name(cluster=w373, "Amplitude"=w379, "omega(0)"=w370, "Gamma"=w371, "phi"=w382, "Q"=w381, "Norm  Ampl"=w380, "z (inf)"=w377) -> (w372:T6)
    }
  }
  "lorentzian out" <- w7
